vi "Write HH Config.vi"(8 "error in (no error)":errorcluster, 10 "HH Config":T1[](array[typedef]) {"ISeq"."Duration [s]" min=0 max=26 format="%#_3p"; "ISeq"."Lower [A]" min=0 max=8 format="%#_3p"; "ISeq"."Upper [A]" min=0 max=8 format="%#_3p"}, 11 "DCM-DSI-HW in":refnum<class "DCM-DSI.lvclass">) -> (0 "error out":errorcluster, 3 "DCM-DSI-HW out":refnum<class "DCM-DSI.lvclass">)   [LabVIEW 2016, in "DCM-DSI.lvclass"]
uses:
  DCM-DSI.lvclass
  <vilib>/Powertrain Controls/Device Drivers/DCM/HH/RT/Config.ctl
  <vilib>/Powertrain Controls/Device Drivers/DCM/HH/RT/Mode.ctl
  <vilib>/Powertrain Controls/Device Drivers/DCM/HH/RT/ISeq.ctl
  DCM-DSI.lvclass/DCM-DSI.ctl
  <vilib>/Powertrain Controls/Device Drivers/DCM/HH/RT/DCM - RT - HH.lvlib
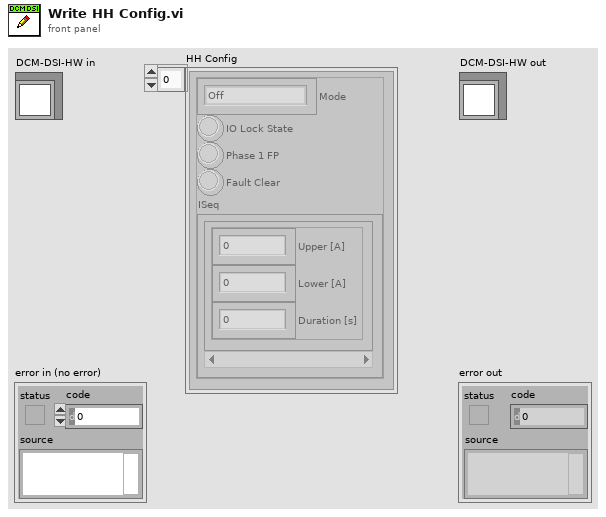
[diagram p1: front panel]
types:
  T1 = typedef "DCM - RT - HH.lvlib/Config.ctl" = cluster{"Mode":T2, "IO Lock State":bool, "Phase 1 FP":bool, "Fault Clear":bool, "ISeq":T3[]}
  T2 = typedef "DCM - RT - HH.lvlib/Mode.ctl" = enum16{"Off", "Lowside", "Highside", "PFI", "Full H", "3-Phase"}
  T3 = typedef "DCM - RT - HH.lvlib/ISeq.ctl" = cluster{"Upper [A]":sgl, "Lower [A]":sgl, "Duration [s]":sgl}
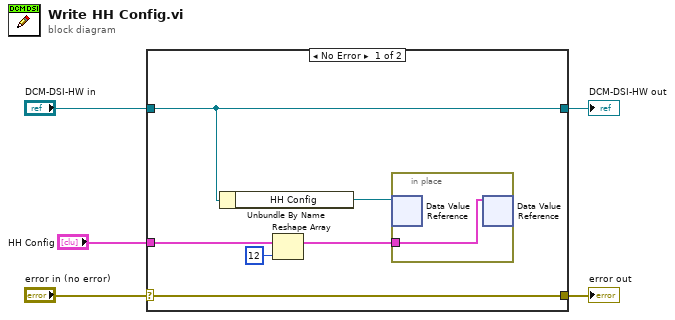
[diagram p0: block diagram]
diagram:
  n1 = case shown="No Error" "error in (no error)" {
    selector: "error in (no error)" -> [w11 w14]
    tunnel: [w11 w14] -> w4
    tunnel: [w9 w13] -> w2
    tunnel: "DCM-DSI-HW in" -> [w9 w13]
    tunnel: "HH Config" -> [w8 _]
    frame No Error {
      n2 = Unbundle By Name(w9) -> ("HH Config"=w10:refnum<data-value>)
      n3 = Reshape Array(w8, 12 ("dimension size")) -> (w7:T1[])
      n4 = in-place {
        in-place-border: w7 -> [w12]
        n5 = in-place-dvr #1(w10) -> ()  [unwired: 2 out]
        n6 = in-place-dvr #1(w12) -> ()  [unwired: 2 out]
      }
    }
    frame Error {
    }
  }
  "error out" <- w4
  "DCM-DSI-HW out" <- w2
